vi "RandomBotLogic.vi"(2 "error in (no error)":errorcluster, 3 "Gameboard":T1) -> (0 "error out":errorcluster, 1 "Selected Index":i8)   [LabVIEW 2020]
uses:
  controls/Gameboard Data.ctl
  controls/Player.ctl
  <vilib>/numeric/Random Number (Range).vi
  <vilib>/numeric/Random Number (Range) I64.vi
  <vilib>/numeric/sub_Random U32.vi
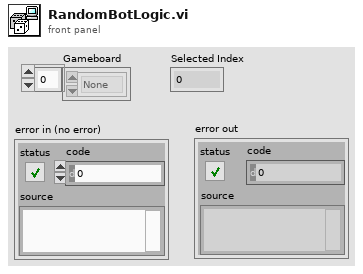
[diagram p1: front panel]
types:
  T1 = typedef "Gameboard Data.ctl" = enum16{"None", "Player 1", "Player 2"}[]
  T2 = typedef "Player.ctl" = enum16{"None", "Player 1", "Player 2"}
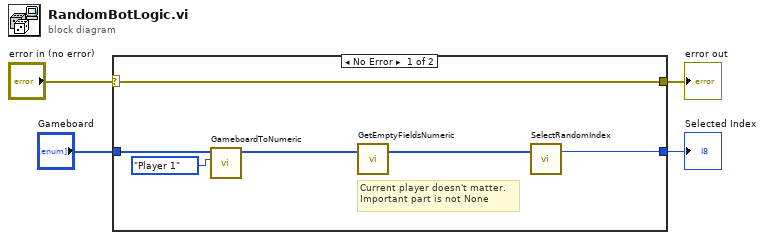
[diagram p0: block diagram]
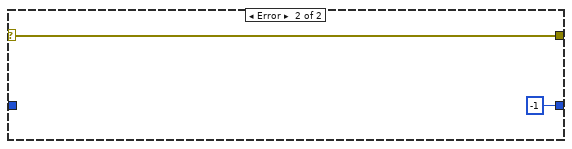
[diagram p2: hidden frame]
diagram:
  n1 = case shown="No Error" "error in (no error)" {
    selector: "error in (no error)" -> [w5 w12]
    tunnel: [w10 i8 -1 ("Selected Index")] -> w4
    tunnel: "Gameboard" -> [w7 _]
    tunnel: [w5 w12] -> w1
    frame No Error {
      # "Current player doesn't matter.\nImportant part is not None"
      n2 = call "GameboardToNumeric.vi"("CurrentPlayer"=Player."Player 1", "Gameboard"=w7) -> ("NumericGameboard"=w8:i8[])  [unwired: 9 in]
      n3 = call "GetEmptyFieldsNumeric.vi"("NumericGameboard"=w8) -> ("Indices"=w9:i8[])  [unwired: 2 in]
      n4 = call "SelectRandomIndex.vi"("Indices"=w9) -> ("Selected Index"=w10:i8)  [unwired: 2 in]
    }
    frame Error {
    }
  }
  "Selected Index" <- w4
  "error out" <- w1
